vi "Create FileHandler.vi"(6 "Flush Timeout (5 s)":dbl=5.0, 8 "error in":errorcluster, 9 "Level":T1, 10 "Name":string, 11 "Filepath":path) -> (0 "error out":errorcluster, 3 "FileHandler out":refnum<class "FileHandler.lvclass">)   [LabVIEW 2020, in "hse-logger.lvlib" / "FileHandler.lvclass"]
doc: "Creates and initializes a new FileHandler object.\n\n____\nHAMPEL SOFTWARE ENGINEERING v2.0.6 (2021-04-15 11:38)"
uses:
  FileHandler.lvclass
  LogLevel.ctl
  hse-logger.lvlib
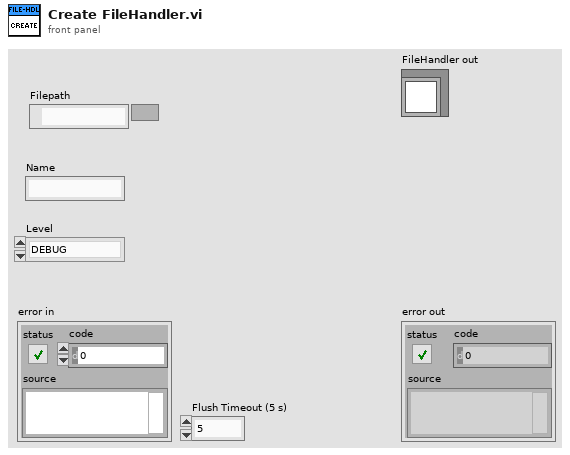
[diagram p1: front panel]
types:
  T1 = typedef "hse-logger.lvlib/LogLevel.ctl" = enum16{"DEBUG", "INFO", "WARNING", "ERROR", "CRITICAL"}
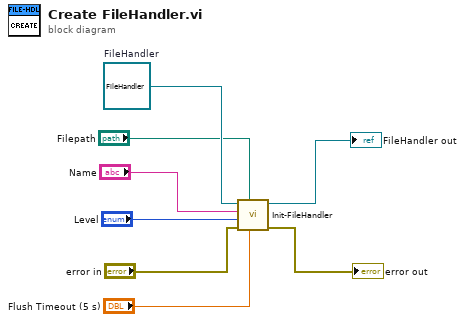
[diagram p0: block diagram]
diagram:
  w8 = refnum<class "FileHandler.lvclass"> refnum  # FileHandler
  n1 = call-dynamic "Init-FileHandler.vi"("Flush Timeout (5 s)"="Flush Timeout (5 s)", "Filepath"="Filepath", "error in"="error in", "Level"="Level", "Name"="Name", "FileHandler"=w8) -> ("error out"=→"error out":errorcluster, "FileHandler out"=→"FileHandler out":refnum<class "FileHandler.lvclass">)  [unwired: 4 in]
